vi "Executer_Create.vi"(0 "reference in":refnum<class "Executer.lvclass">, 2 "Classes":refnum<class>[](array[class]), 5 "error in (no error)":errorcluster) -> (14 "reference out":refnum<class "Executer.lvclass">, 19 "error out":errorcluster)   [LabVIEW 2018, in "Executer.lvclass"]
doc: "This VI creates the Executor class, this class will use the input classes to determine all methods that can be executed, and will determine all information form those methods. \nUse this class to input into a communication class so is can actually execute a method."
uses:
  Executer.lvclass
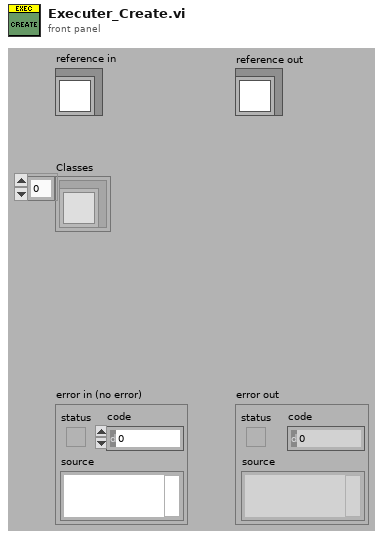
[diagram p1: front panel]
types:
  T1 = typedef "Executer.lvclass/ObjectAttributes.ctl" = cluster{"Executions":T2[]}
  T2 = typedef "Executer.lvclass/ClassExecutionInfo.ctl" = cluster{"Class":refnum<class>, "ClassName":string, "VIExecutionInfo":T3[]}
  T3 = typedef "Executer.lvclass/MethodExecutionInfo.ctl" = cluster{"viRef":refnum<vi>, "MethodName":string, "ControlIndices":i32[], "ClassInIndex":i32, "IndicatorIndices":i32[], "ErrorOutIndex":i32, "ControlTypes":variant[]}
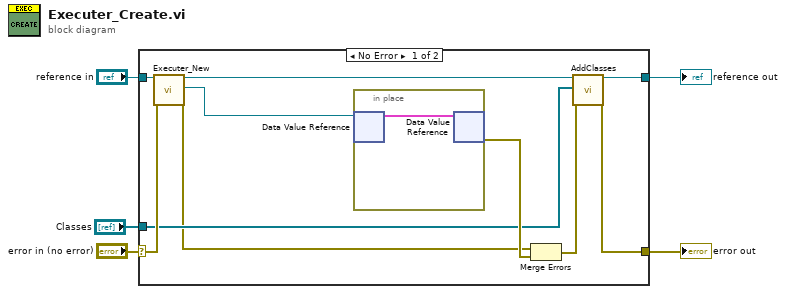
[diagram p0: block diagram]
diagram:
  n1 = case shown="No Error" "error in (no error)" {
    selector: "error in (no error)" -> [w14 w18]
    tunnel: [w10 w18] -> w4
    tunnel: "reference in" -> [w15 w17]
    tunnel: [w8 w17] -> w2
    tunnel: "Classes" -> [w7 _]
    frame No Error {
      n2 = call "Executer_New.vi"("reference in"=w15, "error in (no error)"=w14) -> ("reference out"=w9:refnum<class "Executer.lvclass">, "DVRRefOut"=w12:refnum<data-value>, "error out"=w6:errorcluster)  [unwired: 14 in, 1 out]
      n3 = in-place {
        n4 = in-place-dvr #1(w12) -> (w16:T1)  [unwired: 1 out]
        n5 = in-place-dvr #1(w16) -> (w13:errorcluster)  [unwired: 1 out]
      }
      n6 = Merge Errors(w6, w13) -> (w11:errorcluster)
      n7 = call-dynamic "AddClasses.vi"("reference in"=w9, "Classes"=w7, "error in (no error)"=w11) -> ("reference out"=w8:refnum<class "Executer.lvclass">, "error out"=w10:errorcluster)  [unwired: 15 in]
    }
    frame Error {
      # "VI-TechBaseTemplate_Simple_6x8x6"
    }
  }
  "error out" <- w4
  "reference out" <- w2
